vi "Unpack Control Key Up.vi"(0 "ControlKeyUpMsg":refnum<class "ControlKeyUpMsg.lvclass">) -> (2 "FocusObj":refnum<vi>, 3 "ScanCode":i16, 4 "Ctl Refnum":refnum<vi>, 6 "Control Label":string, 8 "Time":u32, 13 "PlatMods":T1, 14 "Mods":cluster{"Double Click":bool, "Menu Key":bool})   [LabVIEW 2020, in "MVA Framework.lvlib" / "ActorEvents.lvlib" / "ControlKeyUpMsg.lvclass"]
doc: "<License>\nCopyright © 2017 Composed Systems, LLC | All rights reserved\nwww.composed.io\n\nAuthor: Ethan Stern <ethan.stern@composed.io>\n\nThis software is provided \"AS IS\" WITHOUT WARRANTIES, either express or implied, AND IS FOR EDUCATIONAL PURPOSES ONLY.\n</License>"
uses:
  ControlKeyUpMsg.lvclass
  ControlKeyUpMsg.lvclass/ControlKeyUpMsg.ctl
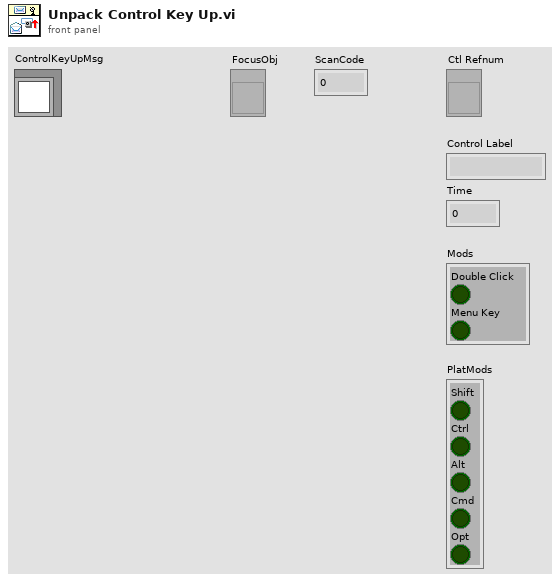
[diagram p1: front panel]
types:
  T1 = cluster{"Shift":bool, "Ctrl":bool, "Alt":bool, "Cmd":bool, "Opt":bool}
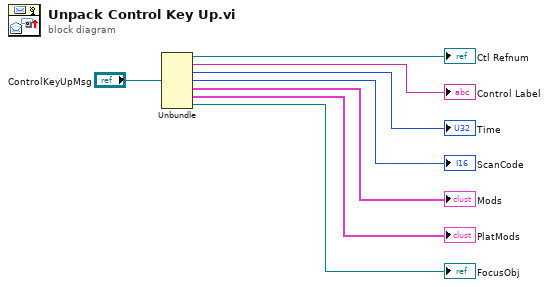
[diagram p0: block diagram]
diagram:
  n1 = Unbundle("ControlKeyUpMsg") -> (→"Ctl Refnum":refnum<vi>, →"Control Label":string, →"Time":u32, →"ScanCode":i16, →"Mods":cluster{"Double Click":bool, "Menu Key":bool}, →"PlatMods":T1, →"FocusObj":refnum<vi>)
